vi "AddMarkers.vi"(10 "Color":u32(colorbox)=32639, 11 "Pixels 3":dbl[][](array[numeric])) -> ()   [LabVIEW 2017]
uses:
  ImageAcquisitionProgram/ImageAcquisitionLibrary/GlobalFrontPanelReferences.vi
  ImageAcquisitionProgram/ImageAcquisitionLibrary/ImageAcquisitionLibrary.lvlib
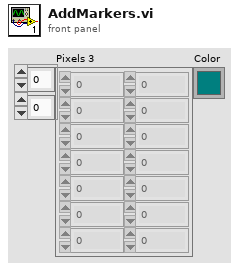
[diagram p1: front panel]
types:
  T1 = typedef "ImageAcquisitionLibrary.lvlib/MarkersArray.ctl" = T2[]
  T2 = typedef "ImageAcquisitionLibrary.lvlib/Marker.ctl" = cluster{"X":dbl, "Color":u32, "Y ":dbl, "Owner":u8}
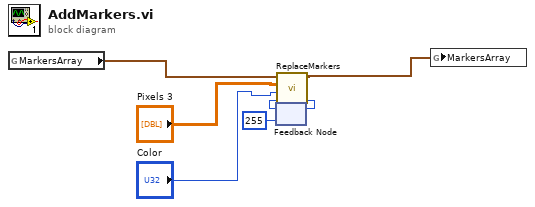
[diagram p0: block diagram]
diagram:
  n1 = global read "GlobalFrontPanelReferences.vi" "MarkersArray"() -> (w6:T1)
  n2 = feedback #1(u8 255 ("Owner Out")) -> (w2:u8)
  n3 = call "ReplaceMarkers.vi"("Owner"=w2, "Color"="Color", "Pixels 3"="Pixels 3", "MarkersArray"=w6) -> ("Owner Out"=w1:u8, "MarkersArray Out"=w5:T1)  [unwired: 6 in]
  n4 = feedback-in #1(w1) -> ()
  n5 = global write "GlobalFrontPanelReferences.vi" "MarkersArray"(w5) -> ()
